vi "Execute.vi"(6 "Error":errorcluster, 7 "Msg":refnum<class "Msg.lvclass">, 11 "Actor":refnum<class "Actor.lvclass">) -> (3 "Actor":refnum<class "Actor.lvclass">, 4 "Error":errorcluster, 5 "Msg":refnum<class "Msg.lvclass">)   [LabVIEW 2020, in "_Template.lvlib" / "{{Msg}}.lvlib" / "Msg.lvclass"]
uses:
  Msg.lvclass
  Msg.lvclass/Msg.ctl
  ActorMsg/ActorMsg.lvclass
  jettl/jettl/Actor/Actor.lvclass
panel:
  # "This front panel should not be manipulated."
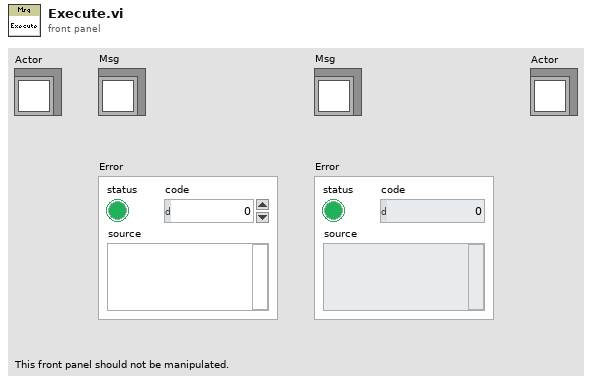
[diagram p1: front panel]
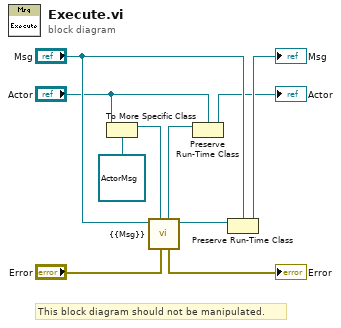
[diagram p0: block diagram]
diagram:
  # "This block diagram should not be manipulated."
  n1 = To More Specific Class(target class=refnum<class "ActorMsg.lvclass"> refnum ("_Template.lvlib:Templates.lvlib:TEMPLATE jettl Msg.lvlib:TEMPLATE jettl Msg.lvclass"), reference="Actor") -> (specific class reference=w7:refnum<class "ActorMsg.lvclass">)  [unwired: 1 in, 1 out]
  n2 = call-dynamic "{{Msg}}.vi"("Error"="Error", "ActorMsg"=w7, "Msg"="Msg") -> ("Msg"=w4:refnum<class "Msg.lvclass">, "Error"=→"Error":errorcluster, "ActorMsg"=w6:refnum<class "ActorMsg.lvclass">)  [unwired: 6 in]
  n3 = Preserve Run-Time Class(object in=w6, 2:"Actor") -> (object out=→"Actor":refnum<class "Actor.lvclass">)  [unwired: 1 in, 1 out]
  n4 = Preserve Run-Time Class(object in=w4, 2:"Msg") -> (object out=→"Msg":refnum<class "Msg.lvclass">)  [unwired: 1 in, 1 out]
